vi "Emballage_BDD_Scann_Datalogic.vi"(0 "COM Réservés":refnum<visa-resource-name>[](array[refnum]), 5 "error in (no error)":errorcluster) -> (14 "COM Array":refnum<visa-resource-name>, 15 "reponse":string[](array[string]), 17 "Nombre de Data trouvés":i32, 18 "ms":u32, 19 "error out":errorcluster)   [LabVIEW 2020]
uses:
  Modules/FS/60_FS_Controles/60_FS_SetGet.ctl
panel:
  out "Com libres":refnum<visa-resource-name>[](array[refnum])
  out "Valide?":bool
  out "Log":string
  out "Interface Information:Interface Description":string
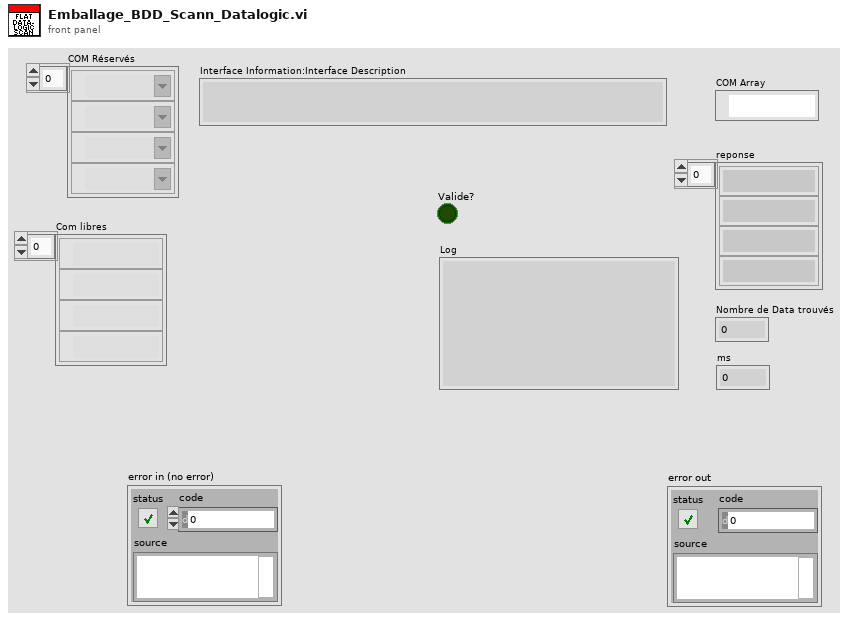
[diagram p1: front panel]
types:
  T1 = typedef "60_FS_SetGet.ctl" = enum16{"set", "get"}
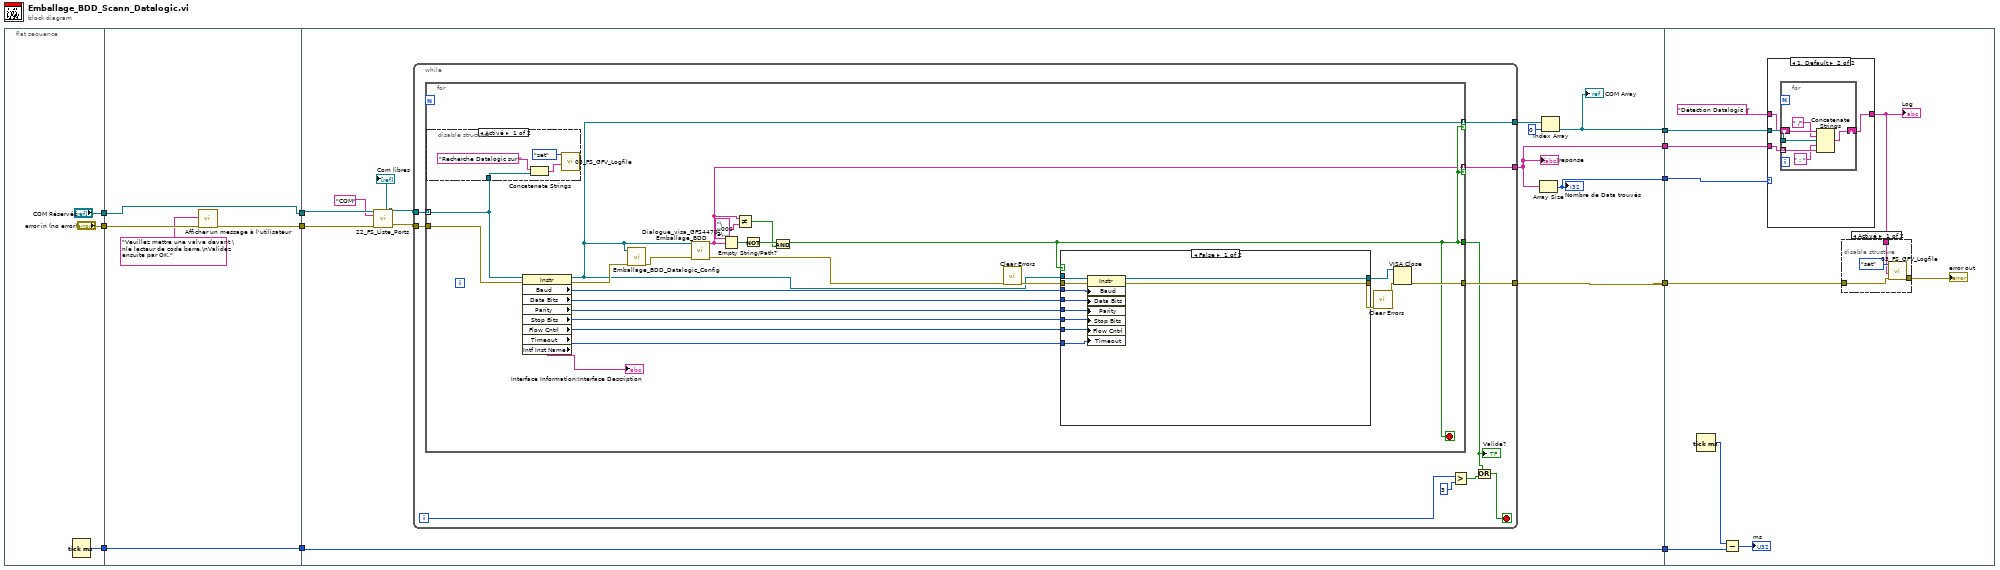
[diagram p0: block diagram]
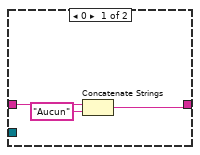
[diagram p5: hidden frame]
diagram:
  n1 = flat-sequence {
    tunnel: [w14] -> w6
    tunnel: ["error in (no error)"] -> w4
    tunnel: ["COM Réservés"] -> w2
    tunnel: w6 -> [w19]
    tunnel: [w19] -> w5
    tunnel: w4 -> [w18]
    tunnel: [w17] -> w3
    tunnel: w2 -> [w15]
    tunnel: [w15] -> w1
    tunnel: w5 -> [w30]
    tunnel: [w30] -> w11
    tunnel: w3 -> [w20]
    tunnel: [w31] -> w10
    tunnel: w1 -> [w29]
    tunnel: [w22] -> w9
    tunnel: [w24] -> w8
    tunnel: [w23] -> w7
    tunnel: w11 -> [w90]
    tunnel: w10 -> [w88]
    tunnel: w9 -> [w87]
    tunnel: w8 -> [w86]
    tunnel: w7 -> [w84]
    frame #0 {
      n2 = Tick Count (ms)() -> (millisecond timer value=w14:u32)
    }
    frame #1 {
      n3 = call "Afficher un message à l'utilisateur"("error in (no error)"=w18, "Message"="Veuillez mettre une valve devant \nle lecteur de code barre.\nValidez ensuite par OK." ("message")) -> ("error out"=w17:errorcluster)  [unwired: 8 in, 1 out]
    }
    frame #2 {
      n4 = call "22_FS_Liste_Ports.vi"("error in (no error)"=w20, "Filtre (sans \"*\")"="COM" ("Filtre (sans \"*\")"), "COM Réservés"=w29) -> ("error out"=w27:errorcluster, "Com libres"=w26:refnum<visa-resource-name>[])  [unwired: 7 in]
      "Com libres" <- w26
      n5 = while {
        tunnel: [w41] -> w31
        tunnel: w27 -> [w40]
        tunnel: w26 -> [w39]
        tunnel: [w38] -> w25
        tunnel: [w37] -> w24
        i -> [w35]
        stop <- w36 stop-if-true
        n6 = for {
          tunnel: [w46] -> w38 mode=indexing if=w45
          tunnel: [w65] -> w41
          tunnel: [w44] -> w37 mode=indexing if=w45
          tunnel: w40 -> [w57]
          tunnel: w39 -> [w56] mode=indexing
          tunnel: [w45] -> w32
          stop <- w45 stop-if-true
          n7 = disable-structure shown="Activé" {
            disable-tunnel: w56 -> [w69 _]
            frame Enabled {
              n8 = Concatenate Strings("Recherche Datalogic sur " ("Chaîne"), w69) -> (w67:string)
              n9 = call "03_FS_GFV_Logfile.vi"("Chaîne"=w67, "States"=60_FS_SetGet."set") -> ()  [unwired: 8 in, 2 out]
            }
            frame Disabled {
            }
          }
          n10 = property class="Instr"(reference=w56, error in=w57) -> (reference out=w46:refnum<visa-resource-name>, error out=w47:errorcluster, "Baud"=w64:u32, "Data Bits"=w63:u16, "Parity"=w62:u16, "Stop Bits"=w61:u16, "Flow Cntrl"=w60:u16, "Timeout"=w59:u32, "Intf Inst Name"=→"Interface Information:Interface Description":string)
          n11 = call "Emballage_BDD_Datalogic_Config.vi"("error in (no error)"=w47, "VISA resource name"=w46) -> ("error out"=w48:errorcluster)  [unwired: 9 in]
          n12 = call "Dialogue_visa_GFS4470_Emballage_BDD.vi"("entrée d'erreur (pas d'erreur)"=w48, "nom de ressource VISA"=w46) -> ("error out"=w51:errorcluster, "buffer lu"=w44:string)  [unwired: 6 in]
          n13 = Empty String/Path?(string/path=w44) -> (empty?=w50:bool)
          n14 = Not Equal?(x=w44, y="\u0002\u0018\r\n") -> (x != y?=w43:bool)
          n15 = Not(x=w50) -> (.not. x?=w49:bool)
          n16 = And(x=w49, y=w43) -> (x .and. y?=w45:bool)
          n17 = call <vilib>:"Clear Errors.vi"("error in (no error)"=w51) -> ("error out"=w52:errorcluster)  [unwired: 5 in, 1 out]
          n18 = case shown="False" w45 {
            tunnel: w52 -> [w79 w81]
            tunnel: [w78 w81] -> w53
            tunnel: w64 -> [w77 _]
            tunnel: w63 -> [w76 _]
            tunnel: w62 -> [w75 _]
            tunnel: w61 -> [w74 _]
            tunnel: w60 -> [w73 _]
            tunnel: w59 -> [w72 _]
            tunnel: [w71 w80] -> w55
            tunnel: w46 -> [w70 w80]
            frame False {
              n19 = property class="Instr"(reference=w70, error in=w79, "Baud"=w77, "Data Bits"=w76, "Parity"=w75, "Stop Bits"=w74, "Flow Cntrl"=w73, "Timeout"=w72) -> (reference out=w71:refnum<visa-resource-name>, error out=w78:errorcluster)
            }
            frame True {
            }
          }
          n20 = call <vilib>:"Clear Errors.vi"("error in (no error)"=w53) -> ("error out"=w54:errorcluster)  [unwired: 5 in, 1 out]
          n21 = VISA Close(VISA resource name=w55, error in (no error)=w54) -> (error out=w65:errorcluster)
        }
        "Valide?" <- w32
        n22 = Greater?(x=w35, y=3) -> (0:w33:bool)
        n23 = Or(x=w32, y=w33) -> (x .or. y?=w36:bool)
      }
      "reponse" <- w24
      n24 = Array Size(array=w24) -> (size(s)=w23:i32)
      "Nombre de Data trouvés" <- w23
      n25 = Index Array(array=w25, index=0 ("indice")) -> (element=w22:refnum<visa-resource-name>)
      "COM Array" <- w22
    }
    frame #3 {
      n26 = Tick Count (ms)() -> (millisecond timer value=w91:u32)
      n27 = Subtract(x=w91, y=w90) -> (x-y=→"ms":u32)
      n28 = case shown="1, Default" w84 {
        tunnel: w87 -> [_ w103]
        tunnel: w86 -> [_ w102]
        tunnel: "Détection Datalogic :" ("Chaîne") -> [w99 w101]
        tunnel: [w97 w100] -> w83
        frame 0 {
          n29 = Concatenate Strings(w99, "Aucun" ("string")) -> (w97:string)
        }
        frame 1, Default {
          n30 = for {
            tunnel: w103 -> [w108]
            tunnel: w102 -> [w106] mode=indexing
            shift-right: [w107] -> w100
            shift-left: w101 -> [w109]
            n31 = Concatenate Strings(w109, " /" ("string"), w108, " : " ("string"), w106) -> (w107:string)
          }
        }
      }
      "Log" <- w83
      n32 = disable-structure shown="Activé" {
        disable-tunnel: [w94 w96] -> w82
        disable-tunnel: w88 -> [w93 w96]
        disable-tunnel: w83 -> [w92 _]
        frame Enabled {
          n33 = call "03_FS_GFV_Logfile.vi"("error in"=w93, "Chaîne"=w92, "States"=60_FS_SetGet."set") -> ("error out"=w94:errorcluster)  [unwired: 7 in, 1 out]
        }
        frame Disabled {
        }
      }
      "error out" <- w82
    }
  }
